vi "test Error Word Bits Checker.vi"(8 "error in":errorcluster, 11 "TestCase in":refnum<class "Import.lvclass">=refnum) -> (0 "error out":errorcluster, 3 "TestCase out":refnum<class "Import.lvclass">)   [LabVIEW 2024, in "Import.lvclass"]
uses:
  Import.lvclass
  <vilib>/NI/NI VeriStand Encoding and Decoding/Encoding.ctl
  <vilib>/NI/NI VeriStand Encoding and Decoding/Encoding and Decoding.lvlib
  Shared/Parameter Definition.ctl
  Shared/VS Channel Definition for Parameter.ctl
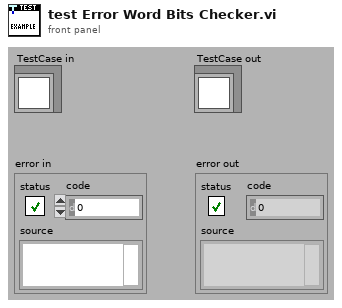
[diagram p1: front panel]
types:
  T1 = cluster{"start bit":i32[], "num bits":i32[], "error text in":string}[]
  T2 = typedef "VS Channel Definition for Parameter.ctl" = cluster{"name":string, "default value":dbl, "unit":string, "Parameter":T3}
  T3 = typedef "Parameter Definition.ctl" = cluster{"start index":i32, "size":i32, "encoding":T4, "signed":bool, "scale multiplier":dbl, "scale offset":dbl}
  T4 = typedef "Encoding and Decoding.lvlib/Encoding.ctl" = enum16{"BNR", "BCD", "Discrete"}
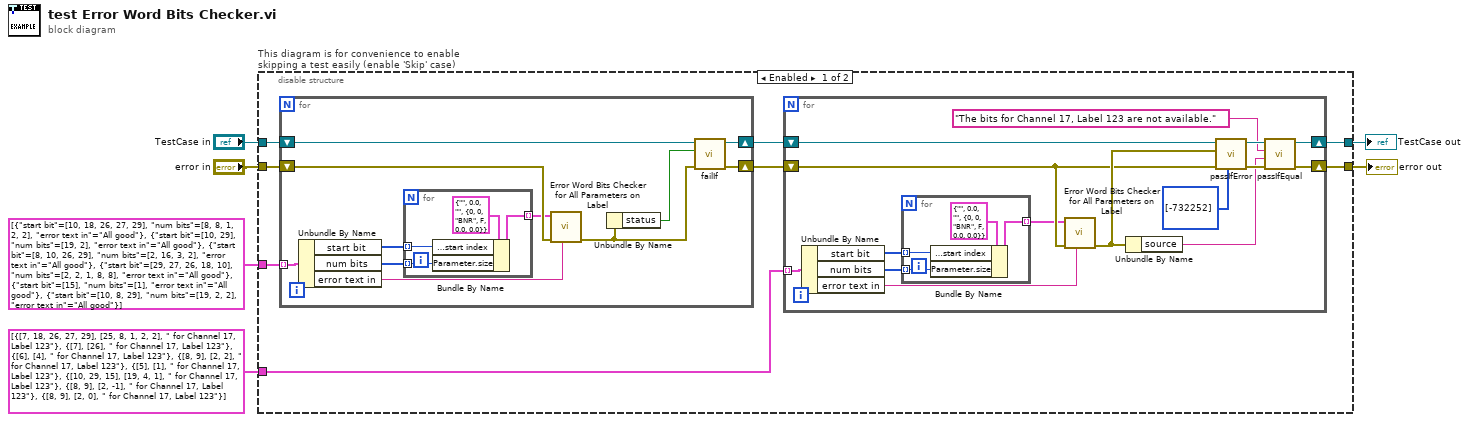
[diagram p0: block diagram]
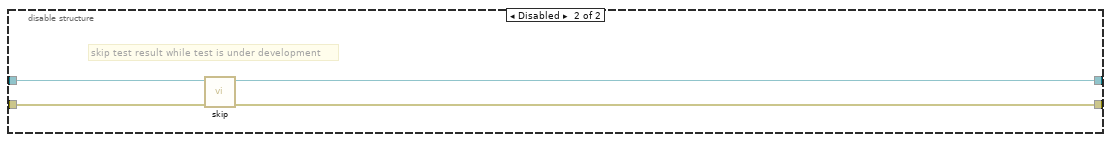
[diagram p2: hidden frame]
diagram:
  n1 = disable-structure "This diagram is for convenience to enable skipping a test easily (enable 'Skip' case)" shown="Enabled" {
    disable-tunnel: "TestCase in" -> [w14 w52]
    disable-tunnel: [w9 w50] -> w3
    disable-tunnel: [w8 w51] -> w5
    disable-tunnel: "error in" -> [w13 w49]
    disable-tunnel: T1 [{"start bit"=[10, 18, 26, 27, 29], "num bits"=[8, 8, 1, 2, 2], "error text in"="All good"}, {"start bit"=[10, 29], "num bits"=[19, 2], "error text in"="All good"}, {"start bit"=[8, 10, 26, 29], "num bits"=[2, 16, 3, 2], "error text in"="All good"}, {"start bit"=[29, 27, 26, 18, 10], "num bits"=[2, 2, 1, 8, 8], "error text in"="All good"}, {"start bit"=[15], "num bits"=[1], "error text in"="All good"}, {"start bit"=[10, 8, 29], "num bits"=[19, 2, 2], "error text in"="All good"}] -> [w12 _]
    disable-tunnel: T1 [{"start bit"=[7, 18, 26, 27, 29], "num bits"=[25, 8, 1, 2, 2], "error text in"=" for Channel 17, Label 123"}, {"start bit"=[7], "num bits"=[26], "error text in"=" for Channel 17, Label 123"}, {"start bit"=[6], "num bits"=[4], "error text in"=" for Channel 17, Label 123"}, {"start bit"=[8, 9], "num bits"=[2, 2], "error text in"=" for Channel 17, Label 123"}, {"start bit"=[5], "num bits"=[1], "error text in"=" for Channel 17, Label 123"}, {"start bit"=[10, 29, 15], "num bits"=[19, 4, 1], "error text in"=" for Channel 17, Label 123"}, {"start bit"=[8, 9], "num bits"=[2, -1], "error text in"=" for Channel 17, Label 123"}, {"start bit"=[8, 9], "num bits"=[2, 0], "error text in"=" for Channel 17, Label 123"}] -> [w7 _]
    frame Enabled {
      n2 = for {
        shift-right: [w43] -> w10
        shift-left: w14 -> [w44]
        shift-right: [w42] -> w11
        shift-left: w13 -> [w37]
        tunnel: w12 -> [w40] mode=indexing
        n3 = Unbundle By Name(w40) -> ("start bit"=w39:i32[], "num bits"=w38:i32[], "error text in"=w34:string)
        n4 = for {
          tunnel: w39 -> [w47] mode=indexing
          tunnel: w38 -> [w46] mode=indexing
          tunnel: [w45] -> w35 mode=indexing
          n5 = Bundle By Name(cluster=T2 {"name"="", "default value"=0.0, "unit"="", "Parameter"={"start index"=0, "size"=0, "encoding"=enum."BNR", "signed"=FALSE, "scale multiplier"=0.0, "scale offset"=0.0}} ("channel parameter"), "Parameter.start index"=w47, "Parameter.size"=w46) -> (w45:T2)
        }
        n6 = call "Error Word Bits Checker for All Parameters on Label.vi"("error text in"=w34, "error in"=w37, "parameters in"=w35) -> ("error out"=w36:errorcluster)  [unwired: 7 in, 1 out]
        n7 = Unbundle By Name(w36) -> ("status"=w41:bool)
        n8 = call-dynamic "failIf.vi"("error in (no error)"=w36, "fail"=w41, "TestCase in"=w44) -> ("error out"=w42:errorcluster, "TestCase out"=w43:refnum<class "Import.lvclass">)  [unwired: 7 in]
      }
      n9 = for {
        shift-right: [w24] -> w9
        shift-left: w10 -> [w29]
        shift-right: [w25] -> w8
        shift-left: w11 -> [w20]
        tunnel: w7 -> [w17] mode=indexing
        n10 = Unbundle By Name(w17) -> ("start bit"=w18:i32[], "num bits"=w19:i32[], "error text in"=w15:string)
        n11 = for {
          tunnel: w18 -> [w32] mode=indexing
          tunnel: w19 -> [w31] mode=indexing
          tunnel: [w30] -> w16 mode=indexing
          n12 = Bundle By Name(cluster=T2 {"name"="", "default value"=0.0, "unit"="", "Parameter"={"start index"=0, "size"=0, "encoding"=enum."BNR", "signed"=FALSE, "scale multiplier"=0.0, "scale offset"=0.0}} ("channel parameter"), "Parameter.start index"=w32, "Parameter.size"=w31) -> (w30:T2)
        }
        n13 = call "Error Word Bits Checker for All Parameters on Label.vi"("error text in"=w15, "error in"=w20, "parameters in"=w16) -> ("error out"=w21:errorcluster)  [unwired: 7 in, 1 out]
        n14 = Unbundle By Name(w21) -> ("source"=w23:string)
        n15 = call-dynamic "passIfError.vi"("passing error codes (default = any error code)"=i32[] [-732252], "error in (no error)"=w20, "error"=w21, "TestCase in"=w29) -> ("error out"=w27:errorcluster, "TestCase out"=w26:refnum<class "Import.lvclass">)  [unwired: 6 in]
        n16 = call-dynamic "passIfEqual.vi"("error in (no error)"=w27, "y"=w23, "x"="The bits for Channel 17, Label 123 are not available.", "TestCase in"=w26) -> ("error out"=w25:errorcluster, "TestCase out"=w24:refnum<class "Import.lvclass">)  [unwired: 6 in]
      }
    }
    frame Disabled {
      # "skip test result while test is under development"
      n17 = call <vilib>:"skip.vi"("error in (no error)"=w49, "TestCase in"=w52) -> ("error out"=w51:errorcluster, "TestCase out"=w50:refnum<class "Import.lvclass">)  [unwired: 8 in]
    }
  }
  "error out" <- w5
  "TestCase out" <- w3
